vi "6 Comp Balance.vi"() -> (0 "DAQ Error":errorcluster)   [LabVIEW 2021]
uses:
  Sub_vis/Upload Data.ctl
  Globals/Meas_global.vi
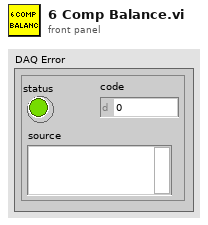
[diagram p1: front panel]
types:
  T1 = typedef "Setup.ctl" = enum16{"Run Program", "Show Setup", "Save Current Setup", "Setup Front Panel"}
  T2 = typedef "Upload Data.ctl" = enum16{"Voltage Array", "Time Trace Cluster"}
  T3 = typedef "Analysis_info_cluster.ctl" = cluster{"Colour":u32, "Inst type":T4, "Inst name":string, "Symbol":string, "Code name":string, "Extra Info":string, "Inst Array":T5, "Extra Titles":string[], "Extra Values":string[], "U":dbl, "u^2":dbl, "u^3":dbl, "u^4":dbl, "Skew_u":dbl, "Kurt_u":dbl, "Sd Error in Mean":dbl, "% u'/U":dbl, "X":dbl, "Y":dbl, "Z":dbl, "Timescale integral Estimate":dbl, "Sd Error in Variance":dbl, "Calib File":path, "Calib Constants":dbl[], "Output Position":bool, "Stats":enum16{"None", "Basic", "Full"}, "Av Sampling Rate":dbl, "Av No of Samples":dbl, "Total Meas Time (s)":dbl, "ADAM Ch Name":string, "Max value":dbl, "Min value":dbl, "Req Sample Rate Hz":dbl, "Sync Delay Time (s)":dbl, "Ch No":i16, "Device":string, "Use Latest Calib":bool, "Port":string, "Metadata Ch Names":string[], "Metadata Ch Values":string[], "Label":string}
  T4 = typedef "Inst_type.ctl" = enum16{"Raw voltage", "Raw with zero offsetting", "Propeller anemometer", "Pressure Transducer", "Pitot-static tube", "Hot wire", "Cross wire 1", "Cross wire 2", "Generic Linear", "Generic Polynomial", "Generic BackPoly", "Fast FID", "Thermocouple", "Cold wire", "Pulsed Wire", "LDA Vel", "LDA Tran time", "LDA Arr time", "Microphone"}
  T5 = typedef "Instrument_Array.ctl" = enum16{"PWA", "LDA", "Analogue"}
  T6 = typedef "Device ID port info.ctl" = cluster{"Ch No":i16[], "Req Sampling Rate":dbl[], "Port":string, "Index":i32[]}
  T7 = typedef "Rendezvous RefNum" = refnum<k1>
  T8 = typedef "Time_Trace_Cluster.ctl" = cluster{"Weighting":dbl[], "Voltage":dbl[], "Eng Values":dbl[]}
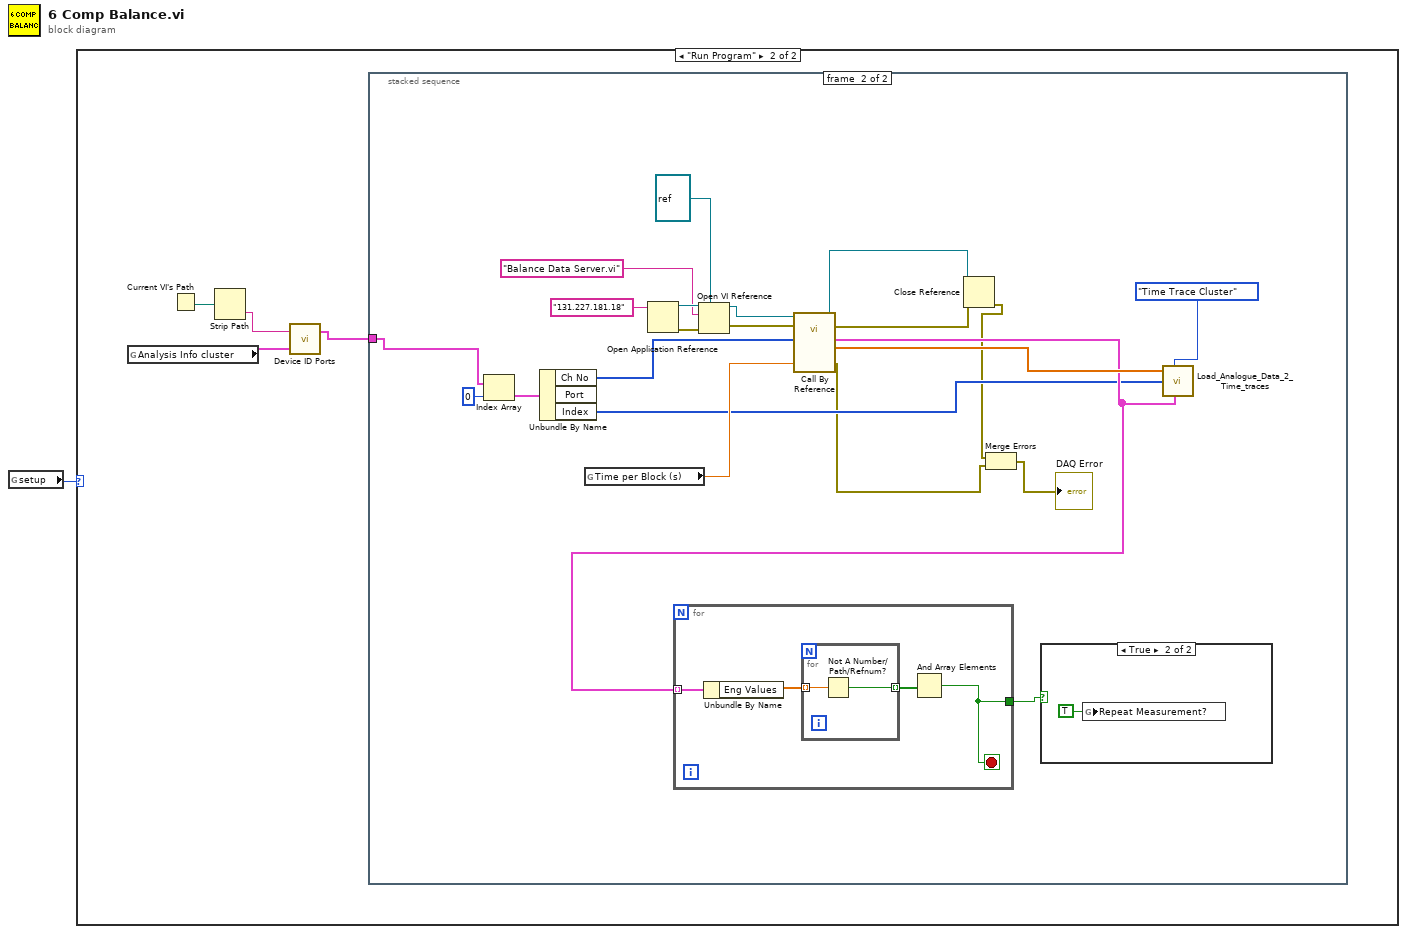
[diagram p0: block diagram]
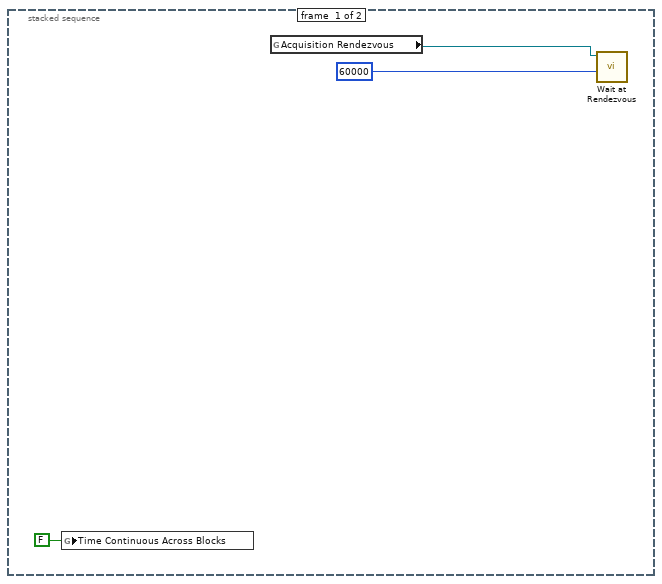
[diagram p3: hidden frame]
diagram:
  n1 = global read "Meas_global.vi" "setup"() -> (w1:T1)
  n2 = case shown="\"Run Program\"" w1 {
    frame Default {
    }
    frame "Run Program" {
      n3 = global read "Meas_global.vi" "Analysis Info cluster"() -> (w5:T3[])
      n4 = Current VI's Path() -> (path=w3:path)
      n5 = Strip Path(path=w3) -> (name=w4:string)  [unwired: 1 out]
      n6 = call "Device ID Ports.vi"("Analysis Info cluster"=w5, "Device ID"=w4) -> ("Device port info"=w2:T6[])  [unwired: 1 out]
      n7 = stacked-sequence {
        tunnel: w2 -> [_ w14]
        frame #0 {
          n8 = global write "Meas_global.vi" "Time Continuous Across Blocks"(FALSE ("Time Continuous across Blocks")) -> ()
          n9 = global read "Meas_global.vi" "Acquisition Rendezvous"() -> (w7:T7)
          n10 = call <vilib>:"Wait at Rendezvous.vi"("ms timeout (-1)"=60000, "rendezvous"=w7) -> ()  [unwired: 3 in, 3 out]
        }
        frame #1 {
          n11 = Index Array(array=w14, index=0) -> (element=w15:T6)
          n12 = Unbundle By Name(w15) -> ("Ch No"=w12:i16[], "Index"=w13:i32[])  [unwired: 1 out]
          n13 = global read "Meas_global.vi" "Time per Block (s)"() -> (w24:dbl)
          n14 = Open Application Reference(11:"131.227.181.18" ("machine name (\"\":  open local reference)")) -> (0:w29:errorcluster, 3:w30:refnum<vi>)  [unwired: 2 in, 1 out]
          n15 = Open VI Reference(type specifier VI Refnum (for type only)=refnum<vi> refnum ("Scout Server"), application reference (local)=w30, vi path="Balance Data Server.vi", error in (no error)=w29) -> (vi reference=w26:refnum<vi>, error out=w25:errorcluster)  [unwired: 2 out]
          n16 = call-by-ref "?"(reference=w26, error in=w25, "Time per Block (s)"=w24, "Ch No"=w12) -> (reference out=w23:refnum<vi>, error out=w22:errorcluster, "DAQ Error"=w10:errorcluster, "Av Sampling Rate"=w19:dbl[], "Time Trace"=w18:T8[])  [unwired: 7 in]
          n17 = for {
            tunnel: w18 -> [w35] mode=indexing
            tunnel: [w32] -> w17
            stop <- w32 stop-if-true
            n18 = Unbundle By Name(w35) -> ("Eng Values"=w34:dbl[])
            n19 = for {
              tunnel: w34 -> [w37] mode=indexing
              tunnel: [w36] -> w33 mode=indexing
              n20 = Not A Number/Path/Refnum?(number/path/refnum=w37) -> (NaN/Path/Refnum?=w36:bool)
            }
            n21 = And Array Elements(Boolean array=w33) -> (logical AND=w32:bool)
          }
          n22 = Close Reference(reference=w23, error in (no error)=w22) -> (error out=w11:errorcluster)
          n23 = Merge Errors(w11, w10) -> (→"DAQ Error":errorcluster)
          n24 = case shown="True" w17 {
            frame False {
            }
            frame True {
              n25 = global write "Meas_global.vi" "Repeat Measurement?"(TRUE ("Repeat Measurement?")) -> ()
            }
          }
          n26 = call "Load_Analogue_Data_2_Time_traces.vi"("Sampling Rate (Hz)"=w19, "Mode"=Upload_Data."Time Trace Cluster", "Index"=w13, "Time Trace"=w18) -> ()  [unwired: 3 in]
        }
      }
    }
  }
